vi "Interpolate Y (single).vi"(8 "error in (no error)":errorcluster, 10 "x (0)":dbl, 11 "XY-data":cluster{"X-array":dbl[], "Y-array":dbl[]}) -> (0 "error out":errorcluster, 2 "y":dbl, 3 "XY-data out":cluster{"X-array":dbl[], "Y-array":dbl[]} {"Y-array" format="%.2p"; "X-array" format="%.2p"})   [LabVIEW 2019, in "xy_utilities.lvlib"]
doc: "Shift the zero value of the x array by giving a new fractional x index.\n\nWire data to the data input to determine the polymorphic instance to use or manually select the instance."
uses:
  xy_utilities.lvlib
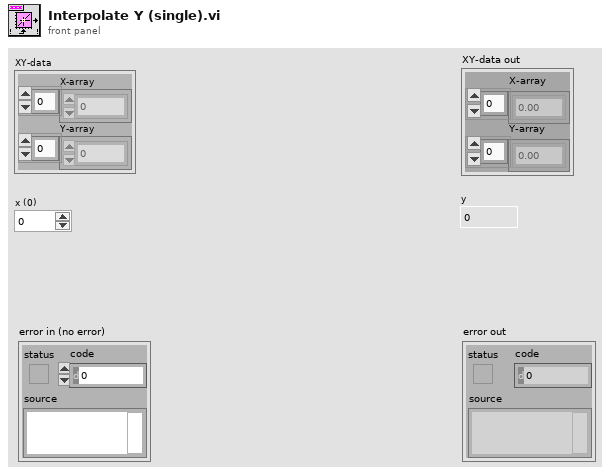
[diagram p1: front panel]
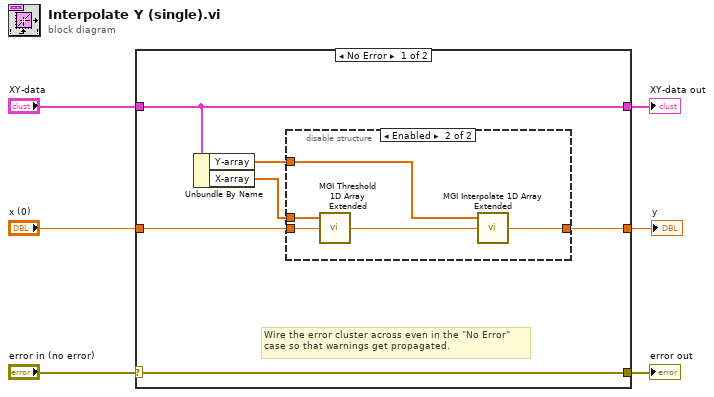
[diagram p0: block diagram]
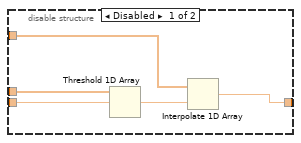
[diagram p2: hidden frame]
diagram:
  n1 = case shown="No Error" "error in (no error)" {
    selector: "error in (no error)" -> [w12 w24]
    tunnel: [w12 w24] -> w5
    tunnel: "XY-data" -> [w10 w23]
    tunnel: [w10 w23] -> w3
    tunnel: "x (0)" -> [w9 _]
    tunnel: [w11 _] -> w1
    frame No Error {
      # "Wire the error cluster across even in the \"No Error\"\ncase so that warnings get propagated."
      n2 = Unbundle By Name(w10) -> ("Y-array"=w8:dbl[], "X-array"=w7:dbl[])
      n3 = disable-structure shown="Enabled" {
        disable-tunnel: [w17 w18] -> w11
        disable-tunnel: w9 -> [w15 w20]
        disable-tunnel: w8 -> [w13 w19]
        disable-tunnel: w7 -> [w14 w21]
        frame Disabled {
          n4 = Threshold 1D Array(2:w15, 3:w14) -> (0:w16:dbl)  [unwired: 1 in]
          n5 = Interpolate 1D Array(1:w16, 2:w13) -> (0:w17:dbl)
        }
        frame Enabled {
          n6 = call "MGI Threshold 1D Array Extended.vi"("Threshold Y"=w20, "Y Value[]"=w21) -> ("Extended Fractional Index"=w22:dbl)  [unwired: 1 in]
          n7 = call "MGI Interpolate 1D Array Extended.vi"("Fractional X"=w22, "Y Value[]"=w19) -> ("ExtendedY"=w18:dbl)  [unwired: 1 in]
        }
      }
    }
    frame Error {
    }
  }
  "error out" <- w5
  "XY-data out" <- w3
  "y" <- w1
